vi "GetSourceRange.vi"(7 "SMU":T2, 8 "Error In":errorcluster, 10 "Source Function":T1, 11 "Kiethley 2602 In":refnum<visa-resource-name>) -> (0 "Error Out":errorcluster, 2 "Range (V or A)":dbl, 3 "Keithley 2602 Out":refnum<visa-resource-name>)   [LabVIEW 2012, in "Keithley-2602.lvlib"]
uses:
  Keithley-2602.lvlib
  Controls/SMU.ctl
  Controls/SourceFunction.ctl
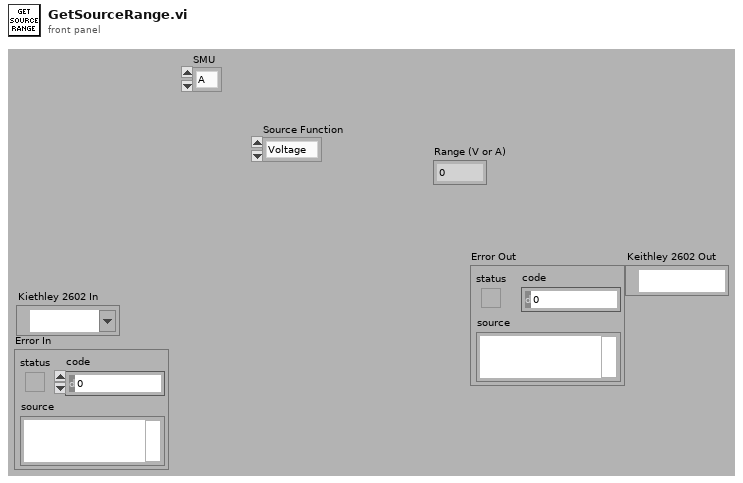
[diagram p1: front panel]
types:
  T1 = typedef "Keithley-2602.lvlib/SourceFunction.ctl" = enum16{"Voltage", "Current"}
  T2 = typedef "Keithley-2602.lvlib/SMU.ctl" = enum16{"A", "B"}
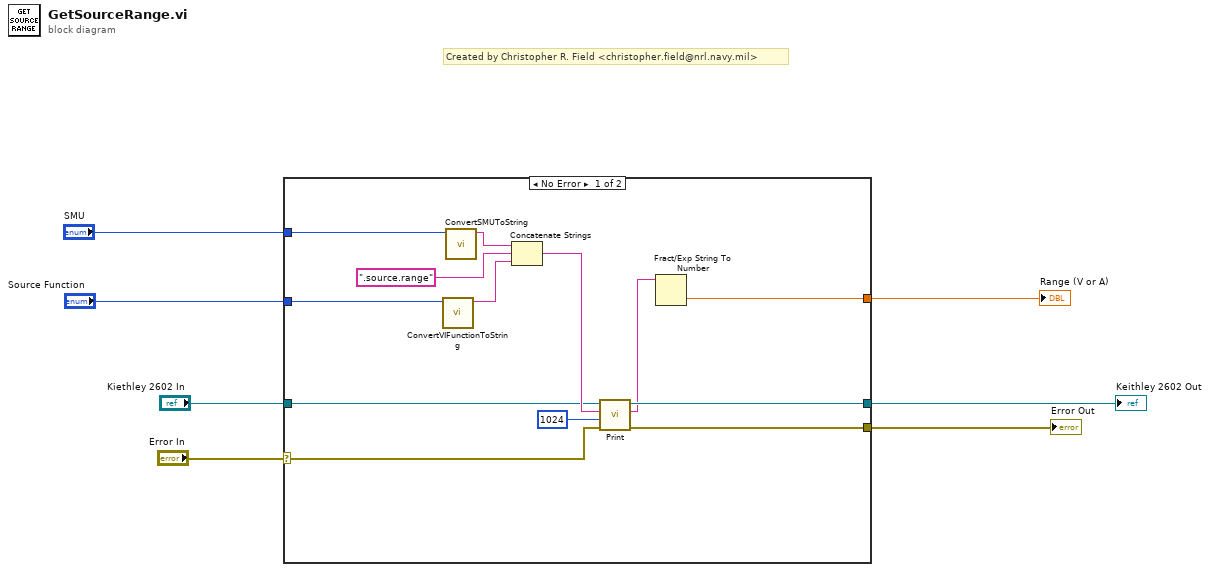
[diagram p0: block diagram]
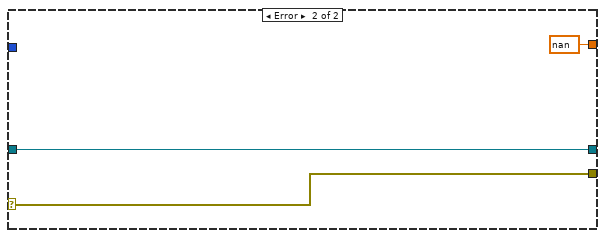
[diagram p2: hidden frame]
diagram:
  # "Created by Christopher R. Field <christopher.field@nrl.navy.mil>"
  n1 = case shown="No Error" "Error In" {
    selector: "Error In" -> [w8 w22]
    tunnel: [w16 w22] -> w7
    tunnel: [w15 w23] -> w6
    tunnel: [w12 nan] -> w5
    tunnel: "Source Function" -> [w11 _]
    tunnel: "SMU" -> [w10 _]
    tunnel: "Kiethley 2602 In" -> [w9 w23]
    frame No Error {
      n2 = call "ConvertVIFunctionToString.vi"("Function"=w11) -> ("Function (v or i)"=w14:string)  [unwired: 10 in]
      n3 = call "ConvertSMUToString.vi"("SMU"=w10) -> ("Channel"=w20:string)  [unwired: 10 in]
      n4 = Concatenate Strings(w20, ".source.range", w14) -> (w18:string)
      n5 = call "Print.vi"("Error In"=w8, "Byte Count"=u32 1024, "Attribute"=w18, "Kiethley 2602 In"=w9) -> ("Error Out"=w16:errorcluster, "Output"=w13:string, "Keithley 2602 Out"=w15:refnum<visa-resource-name>)  [unwired: 5 in]
      n6 = Fract/Exp String To Number(string=w13) -> (number=w12:dbl)  [unwired: 3 in, 1 out]
    }
    frame Error {
    }
  }
  "Error Out" <- w7
  "Keithley 2602 Out" <- w6
  "Range (V or A)" <- w5
